vi "T1.vi"(6 "resolution (ns)":dbl, 9 "pi":dbl[unit], 10 "Gain":dbl, 11 "margin (ns)":i32) -> (2 "Array":dbl[](array[numeric]), 3 "Array size":i32)   [LabVIEW 2015]
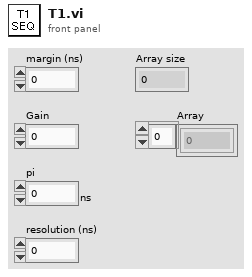
[diagram p1: front panel]
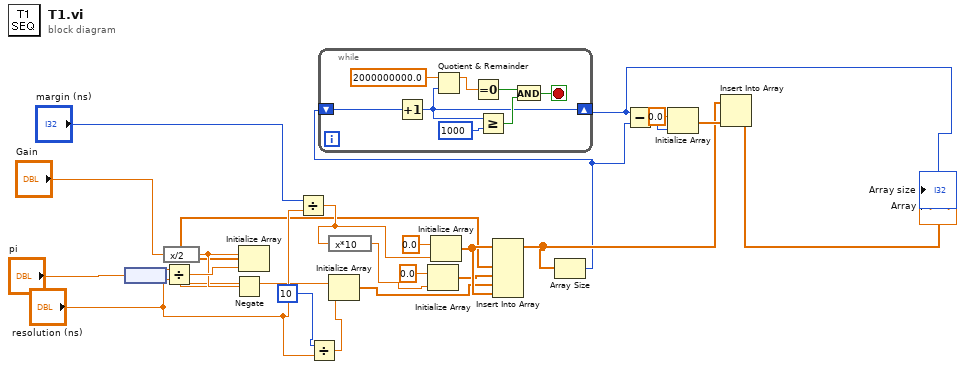
[diagram p0: block diagram]
diagram:
  n1 = node("pi") -> (w11:dbl)
  n2 = expression code="x/2"("Gain") -> (w7:dbl)
  n3 = Divide(x=w11, y="resolution (ns)") -> (x/y=w10:dbl)
  n4 = Negate(x=w7) -> (-x=w2:dbl)
  n5 = Initialize Array(w7, w10) -> (w3:dbl[])
  n6 = Divide(x="margin (ns)", y="resolution (ns)") -> (x/y=w16:dbl)
  n7 = Divide(x=10 ("dimension size"), y="resolution (ns)") -> (x/y=w15:dbl)
  n8 = expression code="x*10"(w16) -> (w17:dbl)
  n9 = Initialize Array(w2, w15) -> (w6:dbl[])
  n10 = Initialize Array(0.0 ("element"), w17) -> (w5:dbl[])
  n11 = Initialize Array(0.0 ("element"), w16) -> (w18:dbl[])
  n12 = Insert Into Array(array=w18, new element #1=w3, new element #2=w5, new element #3=w6, new element #4=w18) -> (w22:dbl[])  [unwired: 1 in]
  n13 = Array Size(array=w22) -> (size(s)=w19:i32)
  n14 = while {
    shift-right: [w27] -> w25
    shift-left: w19 -> [w33]
    stop <- w29 stop-if-true
    n15 = Increment(x=w33) -> (x+1=w27:i32)
    n16 = Quotient & Remainder(x=2000000000.0, y=w27) -> (x-y*floor(x/y)=w31:dbl)  [unwired: 1 out]
    n17 = Equal To 0?(x=w31) -> (x = 0?=w28:bool)
    n18 = Greater Or Equal?(x=w27, y=1000) -> (x >= y?=w30:bool)
    n19 = And(x=w28, y=w30) -> (x .and. y?=w29:bool)
  }
  "Array size" <- w25
  n20 = Subtract(x=w25, y=w19) -> (x-y=w20:i32)
  n21 = Initialize Array(0.0 ("element"), w20) -> (w23:dbl[])
  n22 = Insert Into Array(array=w22, new element=w23) -> (→"Array":dbl[])  [unwired: 1 in]
